vi "List Mousedown Edit.vi"(9 "Row":i32, 10 "Coords":T1, 11 "Listbox in":refnum<vi>) -> ()   [LabVIEW 2019]
uses:
  <vilib>/Utility/miscctls.llb/LVPoint32TypeDef.ctl
  <vilib>/Utility/miscctls.llb/LVRowAndColumnTypeDef.ctl
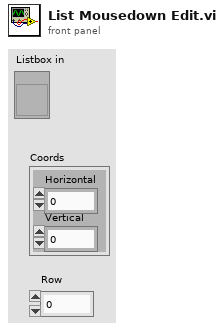
[diagram p1: front panel]
types:
  T1 = typedef "LVPoint32TypeDef.ctl" = cluster{"Horizontal":i32, "Vertical":i32}
  T2 = typedef "LVPositionTypeDef.ctl" = cluster{"Left":i32, "Top":i32}
  T3 = typedef "LVRowAndColumnTypeDef.ctl" = cluster{"Row":i32, "Column":i32}
  T4 = typedef "LVBoundsTypeDef.ctl" = cluster{"Width":u32, "Height":u32}
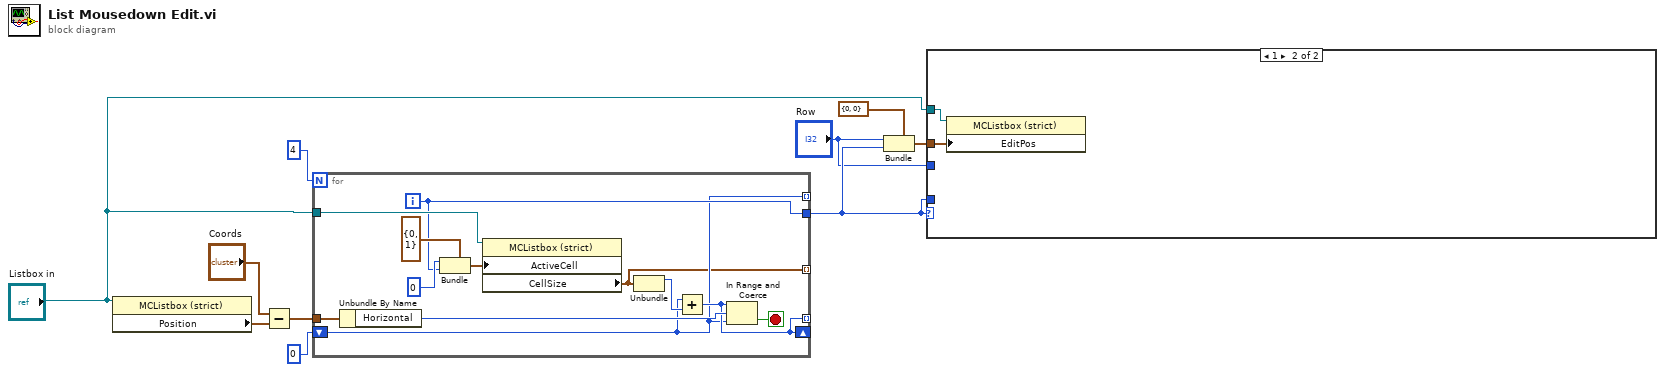
[diagram p0: block diagram]
diagram:
  n1 = property on="Property Node" class="MCListbox (strict)"(reference="Listbox in") -> ("Position"=w3:T2)  [unwired: 1 in, 2 out]
  n2 = Subtract(x="Coords", y=w3) -> (x-y=w5:T1)
  n3 = for {
    N: 4 -> [_]
    tunnel: "Listbox in" -> [w20]
    tunnel: w5 -> [w16]
    shift-right: [w13] -> _
    shift-left: 0 -> [w12]
    tunnel: [w14] -> w9
    tunnel: [w13] -> _ mode=indexing
    tunnel: [w12] -> _ mode=indexing
    tunnel: [w11] -> _ mode=indexing
    i -> [w14]
    stop <- w17 stop-if-true
    n4 = Unbundle By Name(w16) -> ("Horizontal"=w15:i32)
    n5 = Bundle(cluster=T3 {"Row"=0, "Column"=1} ("Active Cell:Active Cell"), "Row"=0, "Column"=w14) -> (w19:T3)
    n6 = property class="MCListbox (strict)"(reference=w20, "ActiveCell"=w19) -> ("CellSize"=w11:T4)  [unwired: 1 in, 2 out]
    n7 = Unbundle(w11) -> ("Width"=w18:u32)  [unwired: 1 out]
    n8 = Add(x=w12, y=w18) -> (x+y=w13:u32)
    n9 = In Range and Coerce(upper limit=w13, x=w15, lower limit=w12) -> (In Range?=w17:bool)  [unwired: 1 out]
  }
  n10 = Bundle(cluster=cluster{"Y":i32, "X":i32} {"Y"=0, "X"=0}, "Y"="Row", "X"=w9) -> (w10:cluster{"Y":i32, "X":i32})
  n11 = case shown="1" w9 {
    tunnel: "Row" -> [_ _]
    tunnel: w9 -> [_ _]
    tunnel: w10 -> [_ w24]
    tunnel: "Listbox in" -> [_ w23]
    frame 0, Default {
    }
    frame 1 {
      n12 = property on="Property Node" class="MCListbox (strict)"(reference=w23, "EditPos"=w24) -> ()  [unwired: 1 in, 2 out]
    }
  }
